vi "Motor Control.vi"() -> ()   [LabVIEW 2017]
uses:
  Control 1.ctl
  Global 1.vi
  DynamixelSDK-3.7.31/labview/dxl_x86_c.lvlib/dxl_x86_c.lvlib
panel:
  in  "Shot":bool
  out "Shot - Act/pas":bool
  out "motor 7":dbl
  out "value : PRO (knob)\npresent position 7":i32(knob)
  out "dynamixel7_id":u8=1
  out "value : PRO (knob)\npresent position 6":i32(knob)
  out "dynamixel6_id":u8=1
  out "motor 1 2":dbl
  out "motor 5":dbl
  out "motor 3 4":dbl
  in  "z value":dbl(slide) scale=29.6..49.6
  out "value : PRO (knob)\npresent position 5":i32(knob)
  out "value : PRO (knob)\npresent position 4":i32(knob)
  out "value : PRO (knob)\npresent position 3":i32(knob)
  out "dynamixel5_id":u8=1
  out "dynamixel4_id":u8=1
  out "dynamixel3_id":T1=1
  out "dynamixel_error":string
  out "dynamixel_comm_result":string
  out "groupread_num":i32
  in  "LEN_PRO_\nPRESENT_POSITION":u16=4
  out "groupwrite_num":i32
  in  "LEN_PRO_\nGOAL_POSITION":u16=4
  out "value : PRO (knob)\npresent position 2":i32(knob)
  in  "dynamixe2_id":u8=2
  in  "device_name":string="COM1"
  out "ADDR_PRO_\nPRESENT_POSITION":u16=611
  out "ADDR_PRO_\nGOAL_POSITION":u16=596
  out "ADDR_PRO_\nTORQUE_ENABLE":u16=562
  out "protocol_version":dbl=2.0
  out "value : PRO (knob)\npresent position 1":i32(knob)
  in  "terminate":bool
  out "port_num":i32
  in  "dynamixel1_id":u8=1
  in  "baud_rate":i32=57600
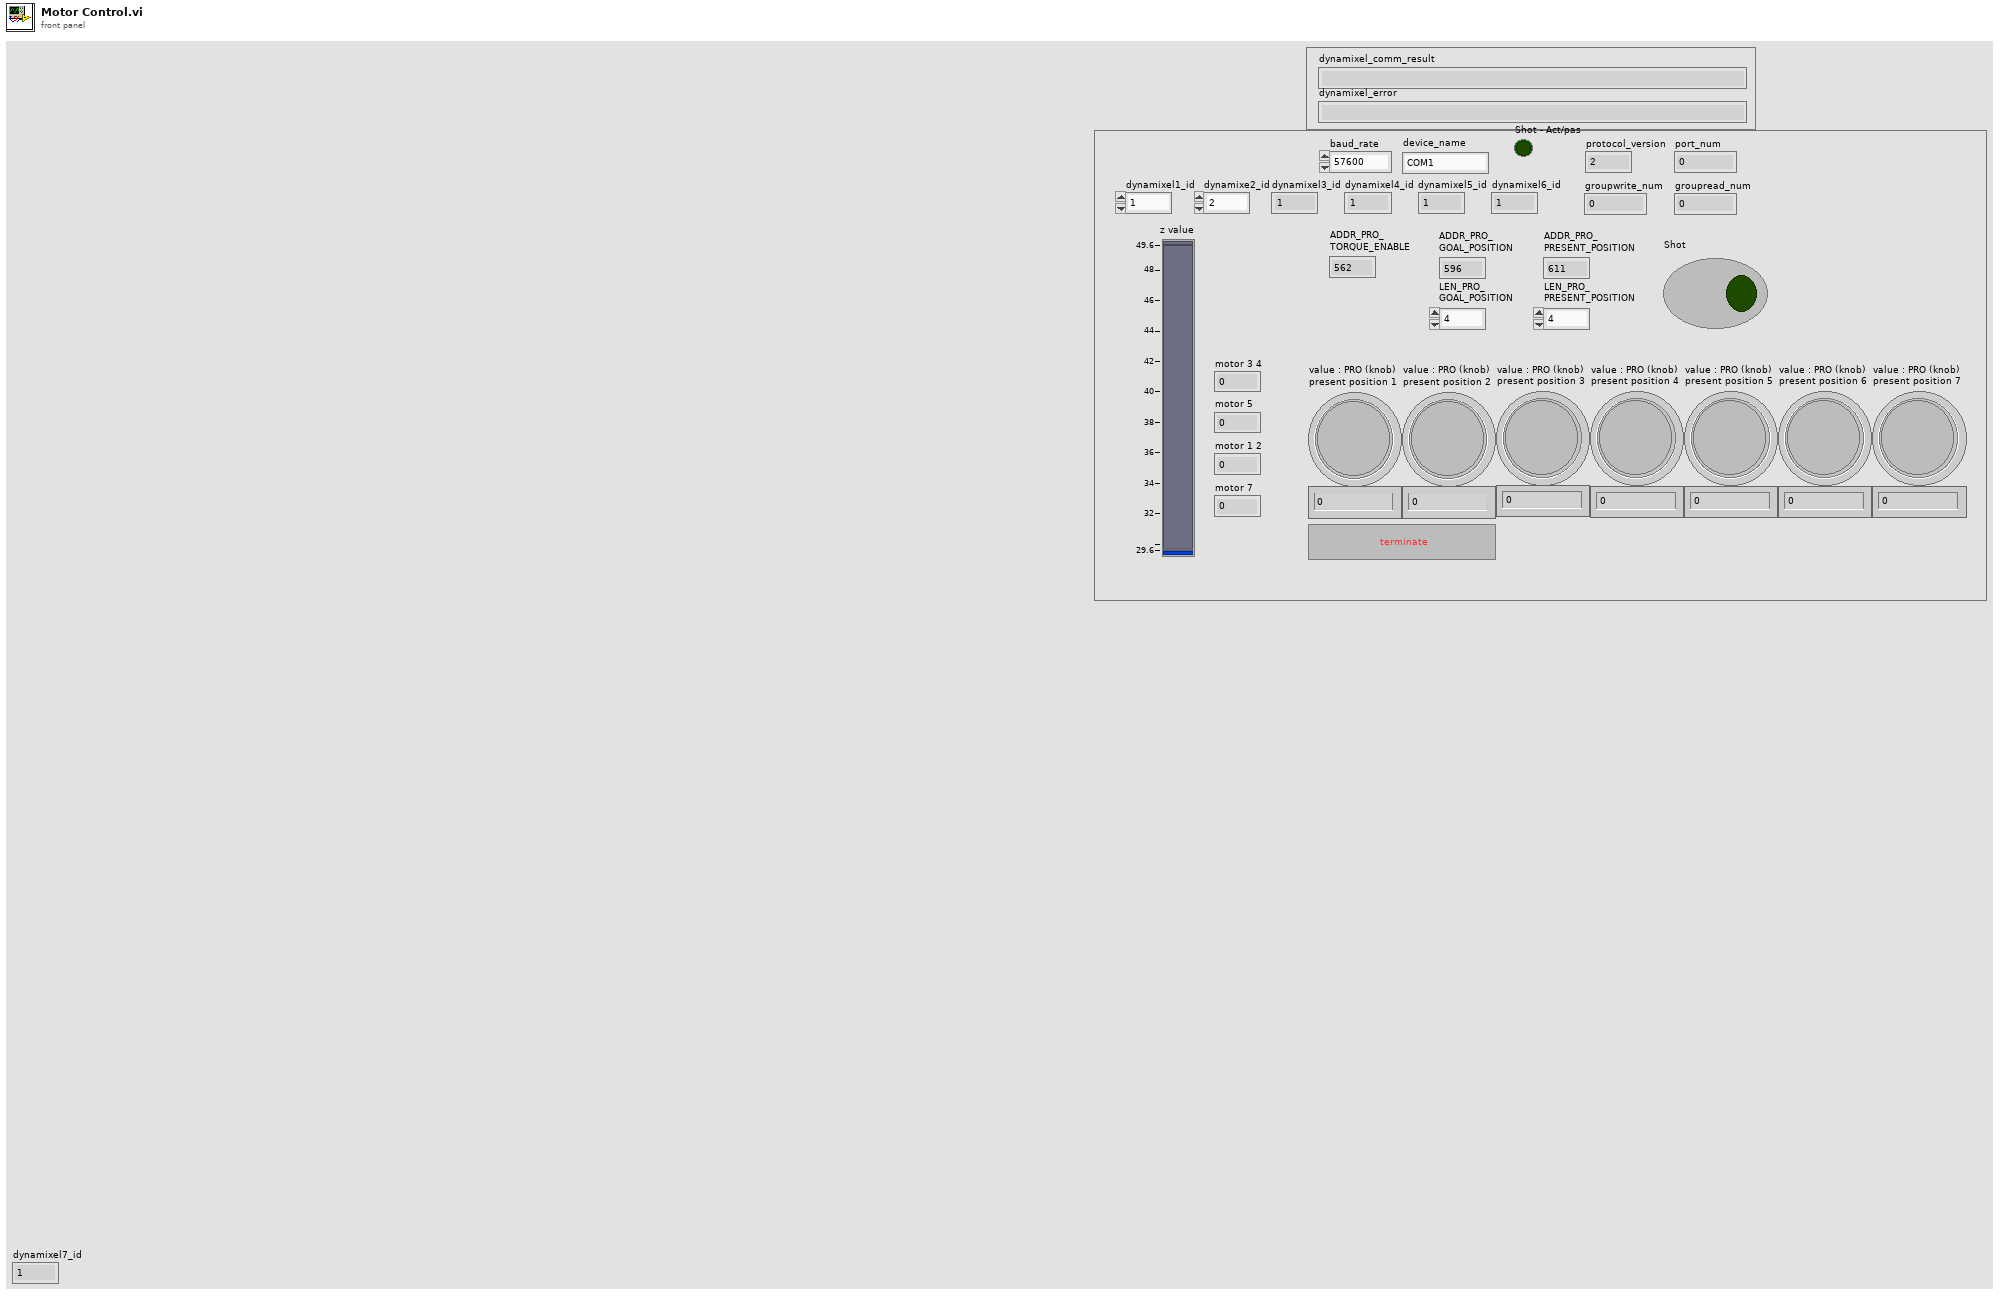
[diagram p1: front panel]
types:
  T1 = typedef "Control 1.ctl" = u8
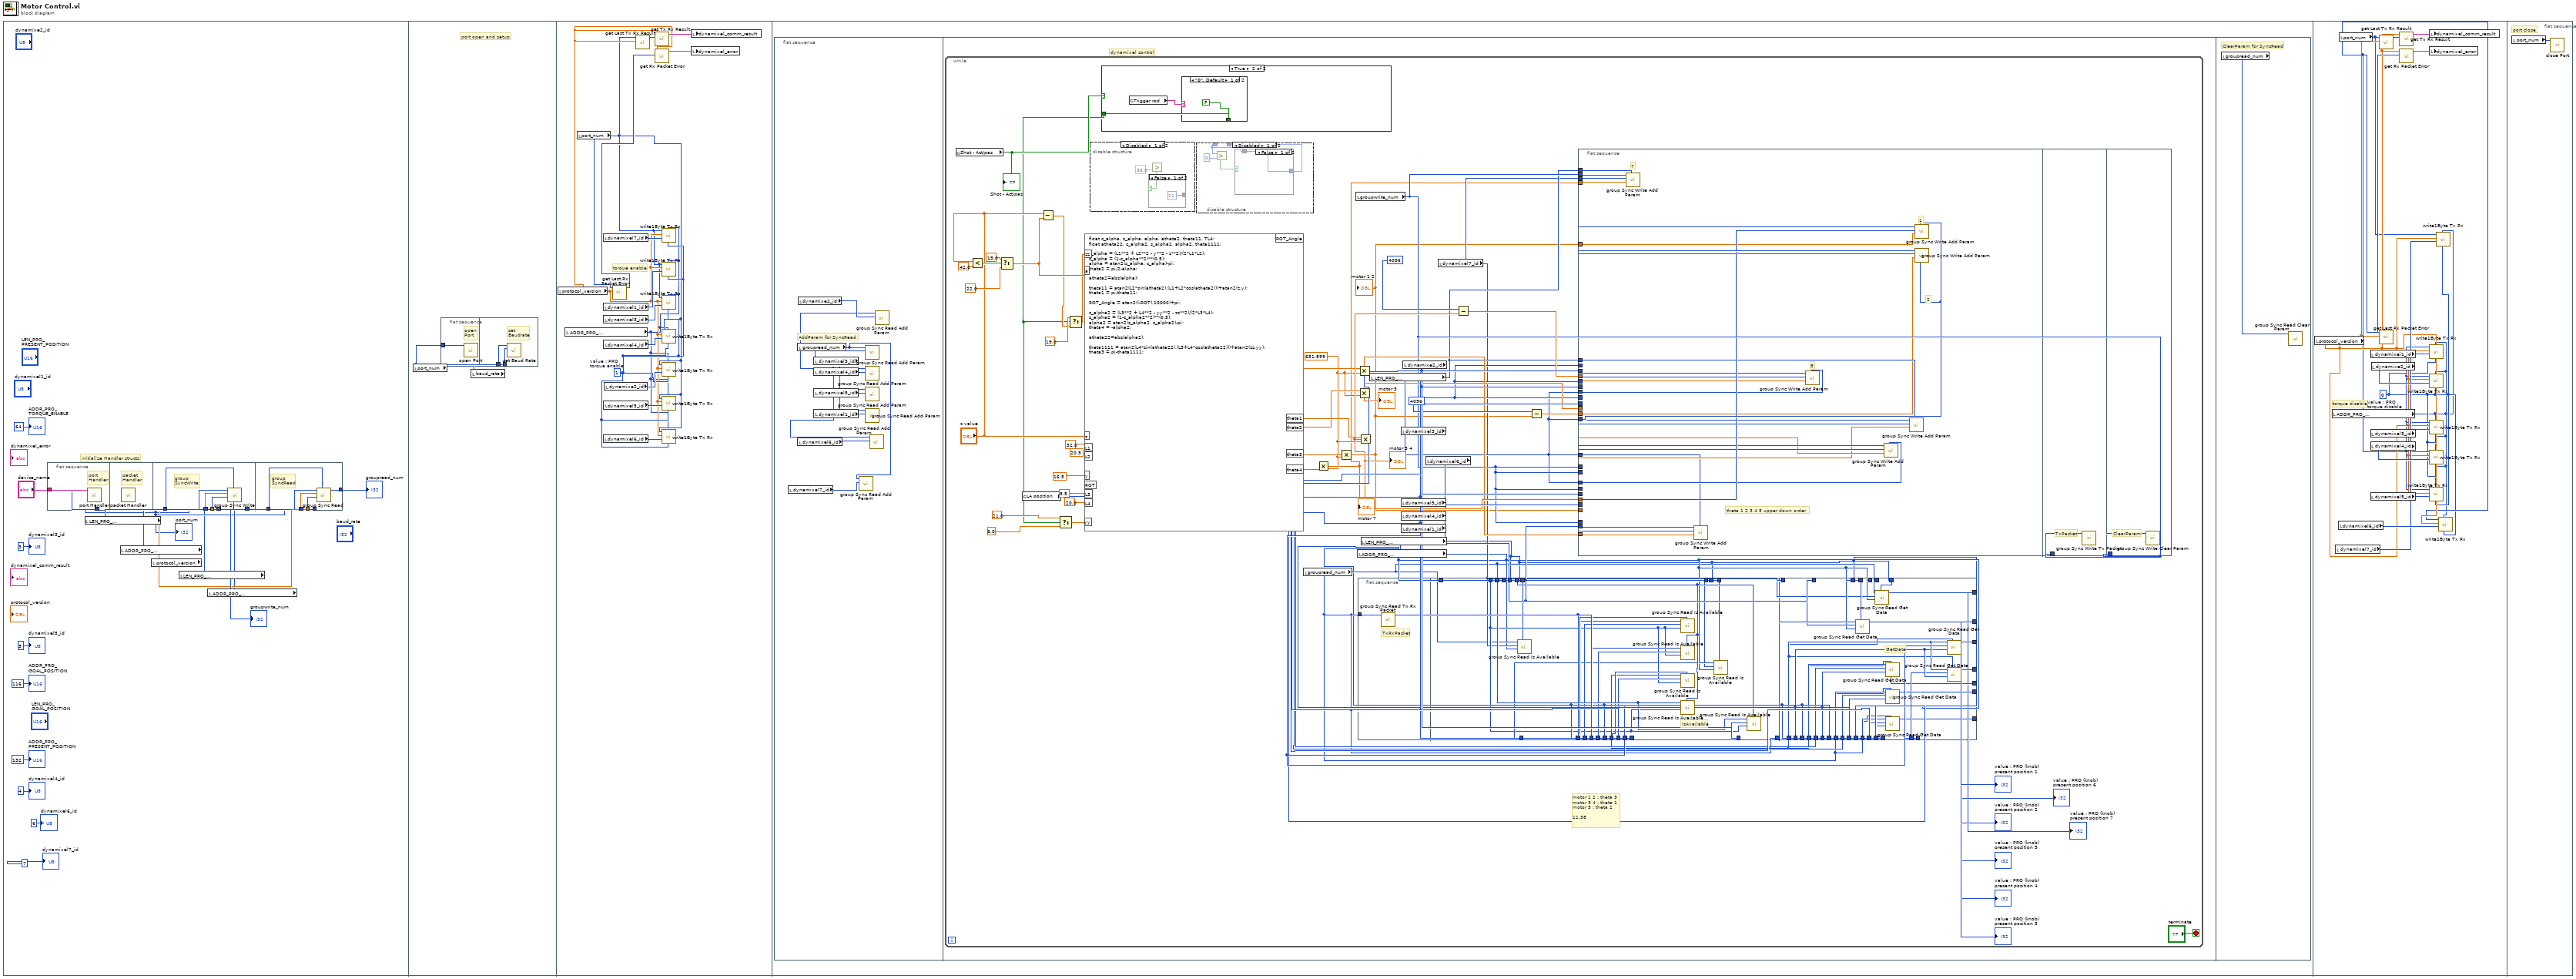
[diagram p0: block diagram]
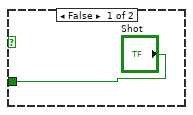
[diagram p2: hidden frame]
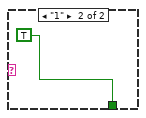
[diagram p3: hidden frame]
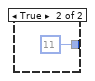
[diagram p4: hidden frame]
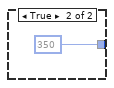
[diagram p6: hidden frame]
diagram:
  n1 = flat-sequence {
    frame #0 {
      # "initialize Handler structs"
      n2 = flat-sequence {
        tunnel: "device_name" -> [w19]
        tunnel: [w18] -> w10
        tunnel: w16 -> [w24]
        tunnel: w15 -> [w23]
        tunnel: w12 -> [w22]
        tunnel: w10 -> [w21]
        tunnel: [w20] -> w14
        tunnel: [w29] -> w13
        tunnel: w12 -> [w28]
        tunnel: w11 -> [w27]
        tunnel: w10 -> [w26]
        tunnel: w9 -> [w25]
        frame #0 {
          # "port\nHandler"
          n3 = call "port Handler.vi"("port_name"=w19) -> ("function return"=w18:i32)  [unwired: 10 in]
        }
        frame #1 {
          # "packet\nHandler"
          n4 = call "packet Handler.vi"() -> ()  [unwired: 12 in]
        }
        frame #2 {
          # "group\nSyncWrite"
          n5 = call "group Sync Write.vi"("data_length"=w24, "start_address"=w23, "protocol_version"=w22, "port_num"=w21) -> ("function return"=w20:i32)  [unwired: 7 in]
        }
        frame #3 {
          # "group\nSyncRead"
          n6 = call "group Sync Read.vi"("data_length"=w25, "start_address"=w27, "protocol_version"=w28, "port_num"=w26) -> ("function return"=w29:i32)  [unwired: 7 in]
        }
      }
      n7 = local read "LEN_PRO_\nGOAL_POSITION"() -> (w16:u16)
      n8 = local read "ADDR_PRO_\nGOAL_POSITION"() -> (w15:u16)
      n9 = local read "protocol_version"() -> (w12:dbl)
      n10 = local read "LEN_PRO_\nPRESENT_POSITION"() -> (w9:u16)
      n11 = local read "ADDR_PRO_\nPRESENT_POSITION"() -> (w11:u16)
      "port_num" <- w10
      "ADDR_PRO_\nTORQUE_ENABLE" <- u16 64 ("ADDR_PRO_\nTORQUE_ENABLE")
      "ADDR_PRO_\nGOAL_POSITION" <- u16 116 ("ADDR_PRO_\nGOAL_POSITION")
      "ADDR_PRO_\nPRESENT_POSITION" <- u16 132 ("ADDR_PRO_\nPRESENT_POSITION")
      "groupwrite_num" <- w14
      "groupread_num" <- w13
      "dynamixel3_id" <- T1 3 ("dynamixel3_id")
      "dynamixel4_id" <- u8 4 ("dynamixel4_id")
      "dynamixel5_id" <- u8 5 ("dynamixel5_id")
      "dynamixel6_id" <- u8 6 ("dynamixel6_id")
      "dynamixel7_id" <- u8 7 ("dynamixel7_id")
    }
    frame #1 {
      # "port open and setup"
      n12 = local read "port_num"() -> (w31:i32)
      n13 = flat-sequence {
        tunnel: w31 -> [w32]
        tunnel: w31 -> [w34]
        tunnel: w30 -> [w33]
        frame #0 {
          # "open\nPort"
          n14 = call "open Port.vi"("port_num"=w32) -> ()  [unwired: 10 in, 1 out]
        }
        frame #1 {
          # "set\nBaudrate"
          n15 = call "set Baud Rate.vi"("baudrate"=w33, "port_num"=w34) -> ()  [unwired: 9 in, 1 out]
        }
      }
      n16 = local read "baud_rate"() -> (w30:i32)
    }
    frame #2 {
      w38 = 1  # value : PRO torque enable
      # "torque enable"
      n17 = local read "protocol_version"() -> (w37:dbl)
      n18 = local read "ADDR_PRO_\nTORQUE_ENABLE"() -> (w35:u16)
      n19 = local read "port_num"() -> (w36:i32)
      n20 = local read "dynamixel7_id"() -> (w39:u8)
      n21 = local read "dynamixel1_id"() -> (w49:u8)
      n22 = local read "dynamixel3_id"() -> (w43:T1)
      n23 = local read "dynamixel4_id"() -> (w42:u8)
      n24 = local read "dynamixel5_id"() -> (w41:u8)
      n25 = local read "dynamixel6_id"() -> (w40:u8)
      n26 = local read "dynamixe2_id"() -> (w48:u8)
      n27 = call "get Last Rx Packet Error.vi"("protocol_version"=w37, "port_num"=w36) -> ("function return"=w46:u8)  [unwired: 9 in]
      n28 = call "get Last Tx Rx Result.vi"("protocol_version"=w37, "port_num"=w36) -> ("function return"=w47:i32)  [unwired: 9 in]
      n29 = call "get Tx Rx Result.vi"("result"=w47, "protocol_version"=w37) -> ("function return"=w45:string)  [unwired: 9 in]
      n30 = call "get Rx Packet Error.vi"("error"=w46, "protocol_version"=w37) -> ("function return"=w44:string)  [unwired: 9 in]
      n31 = call "write1Byte Tx Rx.vi"("data"=w38, "address"=w35, "id"=w39, "protocol_version"=w37, "port_num"=w36) -> ()  [unwired: 7 in]
      n32 = call "write1Byte Tx Rx.vi"("data"=w38, "address"=w35, "id"=w49, "protocol_version"=w37, "port_num"=w36) -> ()  [unwired: 7 in]
      n33 = call "write1Byte Tx Rx.vi"("data"=w38, "address"=w35, "id"=w43, "protocol_version"=w37, "port_num"=w36) -> ()  [unwired: 7 in]
      n34 = call "write1Byte Tx Rx.vi"("data"=w38, "address"=w35, "id"=w42, "protocol_version"=w37, "port_num"=w36) -> ()  [unwired: 7 in]
      n35 = call "write1Byte Tx Rx.vi"("data"=w38, "address"=w35, "id"=w48, "protocol_version"=w37, "port_num"=w36) -> ()  [unwired: 7 in]
      n36 = call "write1Byte Tx Rx.vi"("data"=w38, "address"=w35, "id"=w41, "protocol_version"=w37, "port_num"=w36) -> ()  [unwired: 7 in]
      n37 = call "write1Byte Tx Rx.vi"("data"=w38, "address"=w35, "id"=w40, "protocol_version"=w37, "port_num"=w36) -> ()  [unwired: 7 in]
      n38 = local write "dynamixel_comm_result"(w45) -> ()
      n39 = local write "dynamixel_error"(w44) -> ()
    }
    frame #3 {
      n40 = flat-sequence {
        frame #0 {
          # "AddParam for SyncRead"
          n41 = local read "dynamixel7_id"() -> (w51:u8)
          n42 = local read "groupread_num"() -> (w50:i32)
          n43 = local read "dynamixel6_id"() -> (w52:u8)
          n44 = local read "dynamixe2_id"() -> (w56:u8)
          n45 = local read "dynamixel3_id"() -> (w55:T1)
          n46 = local read "dynamixel4_id"() -> (w54:u8)
          n47 = local read "dynamixel5_id"() -> (w53:u8)
          n48 = local read "dynamixel1_id"() -> (w57:u8)
          n49 = call "group Sync Read Add Param.vi"("id"=w51, "group_num"=w50) -> ()  [unwired: 9 in, 1 out]
          n50 = call "group Sync Read Add Param.vi"("id"=w55, "group_num"=w50) -> ()  [unwired: 9 in, 1 out]
          n51 = call "group Sync Read Add Param.vi"("id"=w54, "group_num"=w50) -> ()  [unwired: 9 in, 1 out]
          n52 = call "group Sync Read Add Param.vi"("id"=w53, "group_num"=w50) -> ()  [unwired: 9 in, 1 out]
          n53 = call "group Sync Read Add Param.vi"("id"=w57, "group_num"=w50) -> ()  [unwired: 9 in, 1 out]
          n54 = call "group Sync Read Add Param.vi"("id"=w52, "group_num"=w50) -> ()  [unwired: 9 in, 1 out]
          n55 = call "group Sync Read Add Param.vi"("id"=w56, "group_num"=w50) -> ()  [unwired: 9 in, 1 out]
        }
        frame #1 {
          # "dynamixel control"
          n56 = while {
            stop <- "terminate" stop-if-true
            w76 = 651.899
            # "motor 1 2 : theta 3\nmotor 3 4 : theta 1\nmotor 5 : theta 2\n\n11.38"
            n57 = global read "Global 1.vi" "Shot - Act/pas"() -> (w59:bool)
            "Shot - Act/pas" <- w59
            n58 = Less?(x="z value", y=42.0) -> (x < y?=w72:bool)
            n59 = Select(t=15.0, s=w72, f=22.0) -> (s? t:f=w69:dbl)
            n60 = global read "Global 1.vi" "LA position"() -> (w86:i32)
            n61 = Subtract(x="z value", y=w69) -> (x-y=w68:dbl)
            n62 = disable-structure shown="Disabled" {
              frame Disabled {
                n63 = Greater?(y=36.0) -> (x=w120:dbl, 0:w118:bool)
                n64 = case shown="False" w118 {
                  tunnel: [11 11] -> _
                  frame False {
                  }
                  frame True {
                  }
                }
              }
              frame Enabled {
              }
            }
            n65 = case shown="True" w59 {
              tunnel: ["Shot" w114] -> w58
              frame False {
              }
              frame True {
                n66 = global read "Global 1.vi" "Trigger rod"() -> (w115:string)
                n67 = case shown="\"0\", Default" w115 {
                  tunnel: [FALSE TRUE] -> w114
                  frame "0", Default {
                  }
                  frame "1" {
                  }
                }
              }
            }
            n68 = Select(t=21.0, s=w58, f=6.0 ("input variable")) -> (s? t:f=w63:dbl)
            n69 = Select(t=19.0 ("y"), s=w58, f=w68) -> (s? t:f=w67:dbl)
            n70 = formula code="float c_alpha, s_alpha, alpha, atheta2, theta11, TL4;\nfloat atheta22, c_alpha2, s_alpha2, alpha2, theta1111;\n\nc_alpha = (L1**2 + L2**2 - y**2 - z**2)/(2*L1*L2);\ns_alpha = (1-c_alpha**2)**(0.5);\nalpha = atan2(s_alpha, c_alpha)-pi;\ntheta2 = pi/2-alpha;\n\natheta2=abs(alpha);\n\ntheta11 = atan2(L2*sin(atheta2),(L1+L2*cos(atheta2)))+atan2(z,y);\ntheta1 = pi-theta11;\n\nROT_Angle = atan2((-ROT),10000)+pi;\n\nc_alpha2 = (L3**2 + L4**2 - yy**2 - zz**2)/(2*L3*L4);\ns_alpha2 = (1-c_alpha2**2)**(0.5);\nalpha2 = atan2(s_alpha2, c_alpha2)-pi;\ntheta4 = -alpha2;\n\natheta22=abs(alpha2);\n\ntheta1111 = atan2(L4*sin(atheta22),(L3+L4*cos(atheta22)))+atan2(zz,yy);\ntheta3 = pi-theta1111;"("z"="z value", "L1"=32.0 ("input variable"), "L2"=20.5 ("input variable"), "y"=16.5 ("input variable"), "ROT"=w86, "L3"=8.5 ("input variable"), "L4"=20.0 ("input variable"), "yy"=w63, "a"=w69, "zz"=w67) -> ("theta1"=w98:dbl, "theta2"=w97:dbl, "theta3"=w99:dbl, "ROT_Angle"=w87:dbl, "theta4"=w77:dbl)
            n71 = disable-structure shown="Disabled" {
              disable-tunnel: [w124 _] -> _
              disable-tunnel: _ -> [w123 _]
              frame Disabled {
                n72 = Greater?(x=w123, y=0) -> (0:w125:bool)
                n73 = case shown="False" w125 {
                  tunnel: [w127 350] -> w124
                  tunnel: w123 -> [w127 _]
                  frame False {
                  }
                  frame True {
                  }
                }
              }
              frame Enabled {
              }
            }
            n74 = local read "groupread_num"() -> (w81:i32)
            n75 = Multiply(x=w77, y=w76) -> (x*y=w75:dbl)
            "motor 7" <- w75
            n76 = Multiply(x=w99, y=w76) -> (x*y=w60:dbl)
            "motor 1 2" <- w60
            n77 = local read "groupwrite_num"() -> (w85:i32)
            n78 = local read "ADDR_PRO_\nPRESENT_POSITION"() -> (w82:u16)
            n79 = Multiply(x=w87, y=w76) -> (x*y=w88:dbl)
            n80 = Multiply(x=w97, y=w76) -> (x*y=w91:dbl)
            "motor 5" <- w91
            n81 = flat-sequence {
              tunnel: w81 -> [w129]
              tunnel: w81 -> [w150]
              tunnel: w111 -> [w149]
              tunnel: w110 -> [w148]
              tunnel: w80 -> [w147]
              tunnel: w80 -> [w146]
              tunnel: w80 -> [w145]
              tunnel: w81 -> [w144]
              tunnel: w81 -> [w143]
              tunnel: w81 -> [w142]
              tunnel: w107 -> [w141]
              tunnel: w106 -> [w140]
              tunnel: w105 -> [w139]
              tunnel: w82 -> [w138]
              tunnel: w81 -> [w137]
              tunnel: w90 -> [w136]
              tunnel: w82 -> [w135]
              tunnel: w80 -> [w134]
              tunnel: w83 -> [w133]
              tunnel: w80 -> [w132]
              tunnel: w81 -> [w131]
              tunnel: w82 -> [w130]
              tunnel: w81 -> [w182]
              tunnel: w111 -> [w181]
              tunnel: w110 -> [w177]
              tunnel: w82 -> [w178]
              tunnel: w80 -> [w176]
              tunnel: [w180] -> w109
              tunnel: [w179] -> w108
              tunnel: w81 -> [w175]
              tunnel: w81 -> [w174]
              tunnel: w81 -> [w173]
              tunnel: w107 -> [w172]
              tunnel: w106 -> [w171]
              tunnel: w105 -> [w170]
              tunnel: w82 -> [w169]
              tunnel: w82 -> [w168]
              tunnel: w82 -> [w167]
              tunnel: w80 -> [w166]
              tunnel: w80 -> [w165]
              tunnel: w80 -> [w164]
              tunnel: [w163] -> w104
              tunnel: [w162] -> w103
              tunnel: [w161] -> w102
              tunnel: w81 -> [w160]
              tunnel: w90 -> [w159]
              tunnel: w82 -> [w158]
              tunnel: w80 -> [w157]
              tunnel: [w156] -> w89
              tunnel: w83 -> [w155]
              tunnel: w82 -> [w154]
              tunnel: w81 -> [w153]
              tunnel: w80 -> [w152]
              tunnel: [w151] -> w79
              frame #0 {
                # "TxRxPacket"
                n82 = call "group Sync Read Tx Rx Packet.vi"("group_num"=w129) -> ()  [unwired: 11 in]
              }
              frame #1 {
                # "IsAvailable"
                n83 = call "group Sync Read Is Available.vi"("data_length"=w132, "address"=w130, "id"=w133, "group_num"=w131) -> ()  [unwired: 7 in, 1 out]
                n84 = call "group Sync Read Is Available.vi"("data_length"=w145, "address"=w138, "id"=w139, "group_num"=w142) -> ()  [unwired: 7 in, 1 out]
                n85 = call "group Sync Read Is Available.vi"("data_length"=w146, "address"=w138, "id"=w140, "group_num"=w143) -> ()  [unwired: 7 in, 1 out]
                n86 = call "group Sync Read Is Available.vi"("data_length"=w147, "address"=w138, "id"=w141, "group_num"=w144) -> ()  [unwired: 7 in, 1 out]
                n87 = call "group Sync Read Is Available.vi"("data_length"=w146, "address"=w138, "id"=w149, "group_num"=w150) -> ()  [unwired: 7 in, 1 out]
                n88 = call "group Sync Read Is Available.vi"("data_length"=w134, "address"=w135, "id"=w136, "group_num"=w137) -> ()  [unwired: 7 in, 1 out]
                n89 = call "group Sync Read Is Available.vi"("data_length"=w146, "address"=w138, "id"=w148, "group_num"=w150) -> ()  [unwired: 7 in, 1 out]
              }
              frame #2 {
                # "GetData"
                n90 = call "group Sync Read Get Data.vi"("data_length"=w157, "address"=w158, "id"=w159, "group_num"=w160) -> ("function return"=w156:u32)  [unwired: 7 in]
                n91 = call "group Sync Read Get Data.vi"("data_length"=w152, "address"=w154, "id"=w155, "group_num"=w153) -> ("function return"=w151:u32)  [unwired: 7 in]
                n92 = call "group Sync Read Get Data.vi"("data_length"=w164, "address"=w167, "id"=w170, "group_num"=w173) -> ("function return"=w161:u32)  [unwired: 7 in]
                n93 = call "group Sync Read Get Data.vi"("data_length"=w165, "address"=w168, "id"=w171, "group_num"=w174) -> ("function return"=w162:u32)  [unwired: 7 in]
                n94 = call "group Sync Read Get Data.vi"("data_length"=w166, "address"=w169, "id"=w172, "group_num"=w175) -> ("function return"=w163:u32)  [unwired: 7 in]
                n95 = call "group Sync Read Get Data.vi"("data_length"=w176, "address"=w178, "id"=w181, "group_num"=w182) -> ("function return"=w180:u32)  [unwired: 7 in]
                n96 = call "group Sync Read Get Data.vi"("data_length"=w176, "address"=w178, "id"=w177, "group_num"=w182) -> ("function return"=w179:u32)  [unwired: 7 in]
              }
            }
            n97 = Multiply(x=w98, y=w76) -> (x*y=w92:dbl)
            "motor 3 4" <- w92
            n98 = local read "LEN_PRO_\nPRESENT_POSITION"() -> (w80:u16)
            n99 = local read "LEN_PRO_\nGOAL_POSITION"() -> (w84:u16)
            n100 = local read "dynamixel3_id"() -> (w107:T1)
            n101 = local read "dynamixel5_id"() -> (w105:u8)
            n102 = local read "dynamixel4_id"() -> (w106:u8)
            n103 = local read "dynamixel1_id"() -> (w111:u8)
            n104 = local read "dynamixe2_id"() -> (w110:u8)
            n105 = local read "dynamixel6_id"() -> (w90:u8)
            n106 = local read "dynamixel7_id"() -> (w83:u8)
            n107 = Subtract(x=4096, y=w92) -> (x-y=w93:dbl)
            n108 = Subtract(x=4096, y=w60) -> (x-y=w94:dbl)
            n109 = flat-sequence {
              tunnel: w84 -> [w209]
              tunnel: w85 -> [w208]
              tunnel: w85 -> [w207]
              tunnel: w111 -> [w206]
              tunnel: w110 -> [w205]
              tunnel: w85 -> [_]
              tunnel: w85 -> [w204]
              tunnel: w85 -> [w203]
              tunnel: w85 -> [w202]
              tunnel: w84 -> [w201]
              tunnel: w84 -> [w200]
              tunnel: w84 -> [w189]
              tunnel: w107 -> [w199]
              tunnel: w106 -> [w198]
              tunnel: w105 -> [w197]
              tunnel: w94 -> [w184]
              tunnel: w60 -> [_]
              tunnel: w93 -> [w194]
              tunnel: w92 -> [w195]
              tunnel: w91 -> [w196]
              tunnel: w90 -> [w193]
              tunnel: w85 -> [w192]
              tunnel: w84 -> [w191]
              tunnel: w88 -> [w190]
              tunnel: w83 -> [w188]
              tunnel: w85 -> [w187]
              tunnel: w84 -> [w186]
              tunnel: w75 -> [w185]
              tunnel: w60 -> [w183]
              tunnel: w85 -> [w210]
              tunnel: w85 -> [w211]
              frame #0 {
                # "5"
                # "2"
                # "1"
                # "7"
                # "theta 1 2 3 4 5 upper down order"
                n110 = call "group Sync Write Add Param.vi"("data_length"=w186, "data"=w185, "id"=w188, "group_num"=w187) -> ()  [unwired: 7 in, 1 out]
                n111 = call "group Sync Write Add Param.vi"("data_length"=w191, "data"=w190, "id"=w193, "group_num"=w192) -> ()  [unwired: 7 in, 1 out]
                n112 = call "group Sync Write Add Param.vi"("data_length"=w189, "data"=w196, "id"=w197, "group_num"=w204) -> ()  [unwired: 7 in, 1 out]
                n113 = call "group Sync Write Add Param.vi"("data_length"=w200, "data"=w195, "id"=w198, "group_num"=w203) -> ()  [unwired: 7 in, 1 out]
                n114 = call "group Sync Write Add Param.vi"("data_length"=w201, "data"=w194, "id"=w199, "group_num"=w202) -> ()  [unwired: 7 in, 1 out]
                n115 = call "group Sync Write Add Param.vi"("data_length"=w209, "data"=w183, "id"=w206, "group_num"=w208) -> ()  [unwired: 7 in, 1 out]
                n116 = call "group Sync Write Add Param.vi"("data_length"=w209, "data"=w184, "id"=w205, "group_num"=w207) -> ()  [unwired: 7 in, 1 out]
              }
              frame #1 {
                # "TxPacket"
                n117 = call "group Sync Write Tx Packet.vi"("group_num"=w210) -> ()  [unwired: 11 in]
              }
              frame #2 {
                # "ClearParam"
                n118 = call "group Sync Write Clear Param.vi"("group_num"=w211) -> ()  [unwired: 11 in]
              }
            }
            "value : PRO (knob)\npresent position 1" <- w109
            "value : PRO (knob)\npresent position 2" <- w108
            "value : PRO (knob)\npresent position 3" <- w104
            "value : PRO (knob)\npresent position 4" <- w103
            "value : PRO (knob)\npresent position 5" <- w102
            "value : PRO (knob)\npresent position 6" <- w89
            "value : PRO (knob)\npresent position 7" <- w79
          }
        }
        frame #2 {
          # "ClearParam for SyncRead"
          n119 = local read "groupread_num"() -> (w212:i32)
          n120 = call "group Sync Read Clear Param.vi"("group_num"=w212) -> ()  [unwired: 11 in]
        }
      }
    }
    frame #4 {
      w214 = 0  # value : PRO torque disable
      # "torque disable"
      n121 = local read "protocol_version"() -> (w216:dbl)
      n122 = local read "ADDR_PRO_\nTORQUE_ENABLE"() -> (w213:u16)
      n123 = local read "dynamixel7_id"() -> (w217:u8)
      n124 = local read "dynamixel6_id"() -> (w218:u8)
      n125 = local read "port_num"() -> (w215:i32)
      n126 = local read "dynamixel1_id"() -> (w227:u8)
      n127 = local read "dynamixel3_id"() -> (w221:T1)
      n128 = local read "dynamixel4_id"() -> (w219:u8)
      n129 = local read "dynamixel5_id"() -> (w220:u8)
      n130 = local read "dynamixe2_id"() -> (w226:u8)
      n131 = call "get Last Tx Rx Result.vi"("protocol_version"=w216, "port_num"=w215) -> ("function return"=w224:i32)  [unwired: 9 in]
      n132 = call "get Last Rx Packet Error.vi"("protocol_version"=w216, "port_num"=w215) -> ("function return"=w225:u8)  [unwired: 9 in]
      n133 = call "get Tx Rx Result.vi"("result"=w224, "protocol_version"=w216) -> ("function return"=w223:string)  [unwired: 9 in]
      n134 = call "get Rx Packet Error.vi"("error"=w225, "protocol_version"=w216) -> ("function return"=w222:string)  [unwired: 9 in]
      n135 = local write "dynamixel_comm_result"(w223) -> ()
      n136 = local write "dynamixel_error"(w222) -> ()
      n137 = call "write1Byte Tx Rx.vi"("data"=w214, "address"=w213, "id"=w227, "protocol_version"=w216, "port_num"=w215) -> ()  [unwired: 7 in]
      n138 = call "write1Byte Tx Rx.vi"("data"=w214, "address"=w213, "id"=w226, "protocol_version"=w216, "port_num"=w215) -> ()  [unwired: 7 in]
      n139 = call "write1Byte Tx Rx.vi"("data"=w214, "address"=w213, "id"=w221, "protocol_version"=w216, "port_num"=w215) -> ()  [unwired: 7 in]
      n140 = call "write1Byte Tx Rx.vi"("data"=w214, "address"=w213, "id"=w219, "protocol_version"=w216, "port_num"=w215) -> ()  [unwired: 7 in]
      n141 = call "write1Byte Tx Rx.vi"("data"=w214, "address"=w213, "id"=w220, "protocol_version"=w216, "port_num"=w215) -> ()  [unwired: 7 in]
      n142 = call "write1Byte Tx Rx.vi"("data"=w214, "address"=w213, "id"=w217, "protocol_version"=w216, "port_num"=w215) -> ()  [unwired: 7 in]
      n143 = call "write1Byte Tx Rx.vi"("data"=w214, "address"=w213, "id"=w218, "protocol_version"=w216, "port_num"=w215) -> ()  [unwired: 7 in]
    }
    frame #5 {
      # "port close"
      n144 = local read "port_num"() -> (w228:i32)
      n145 = call "close Port.vi"("port_num"=w228) -> ()  [unwired: 11 in]
    }
  }
